vi "Test_LaunchHierarchy_StopRootModel_ConfirmOrderlyShutdown.vi"(8 "error in (no error)":errorcluster, 11 "TestCase in":refnum<class "TestLaunchAndShutdown.lvclass">) -> (0 "error out":errorcluster, 3 "TestCase out":refnum<class "TestLaunchAndShutdown.lvclass">)   [LabVIEW 2020, in "TestLaunchAndShutdown.lvclass"]
uses:
  TestLaunchAndShutdown.lvclass
  TestLaunchAndShutdown.lvclass/TestLaunchAndShutdown.ctl
  24bf8875-c008-4f22-9bfa-88e42476d167.vi
  Source/IModel/IModel/IModel.lvclass
  <vilib>/ActorFramework/Actor/Actor.lvclass
  Source/Mediator/Mediator/Mediator.lvclass
  <vilib>/ActorFramework/Stop Msg/Stop Msg.lvclass
  modules/composed-event-logger/Source/String Control Sink/String Control Sink.lvclass
  modules/composed-event-logger/Source/Composed Log/Types/Log Level.ctl
  modules/composed-event-logger/Source/Composed Log/Composed Log.lvlib
  modules/composed-event-logger/Source/String Formats/String Expression Format/String Expression Format.lvclass
  Doubles/RootModelNotifiesWhenStopped/RootModelNotifiesWhenStopped.lvclass
  C:/Git/mva-core/Source/RootModel/RootModel/RootModel.lvclass
  C:/Git/mva-core/Source/IModel/IModel/IModel.lvclass
  C:/Git/mva-core/Source/IObserver/IObserver/IObserver.lvclass
  C:/Program Files (x86)/National Instruments/LabVIEW 2020/vi.lib/ActorFramework/Actor/Actor.lvclass
  C:/Git/mva-core/Test/Doubles/RootModelNotifiesWhenStopped/RootModelNotifiesWhenStopped.lvclass
  9235eea7-0b3a-4059-b346-9cf3c4f5aec4.vi
  C:/Git/mva-core/modules/composed-event-logger/Source/IStringFormat/IStringFormat.lvclass
  C:/Git/mva-core/modules/composed-event-logger/Source/String Formats/String Expression Format/String Expression Format.lvclass
panel:
  in  "String":string
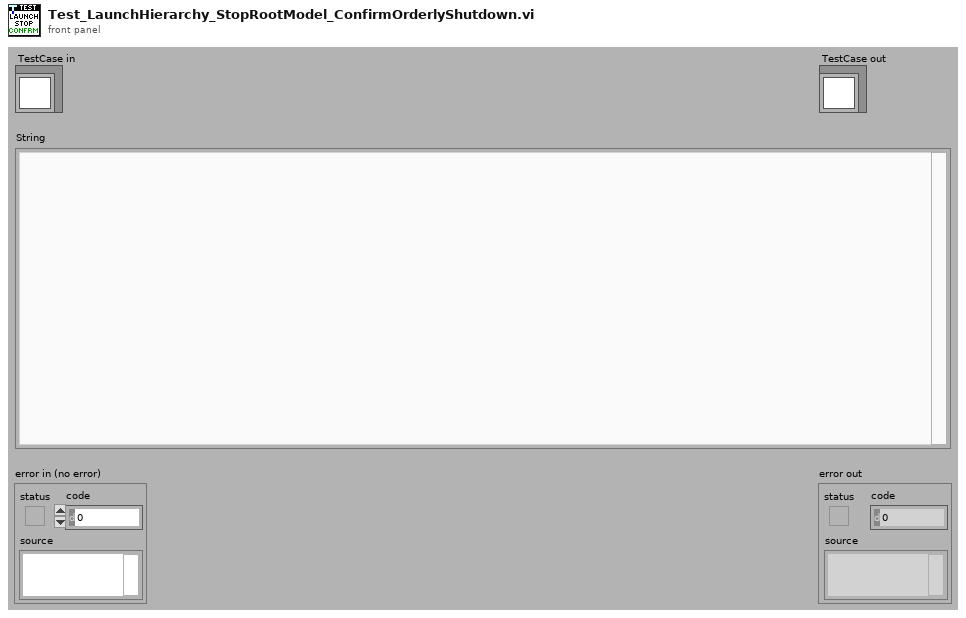
[diagram p1: front panel]
types:
  T1 = typedef "Composed Log.lvlib/Log Level.ctl" = enum16{"Debug", "Info", "Warning", "Error", "Critical"}
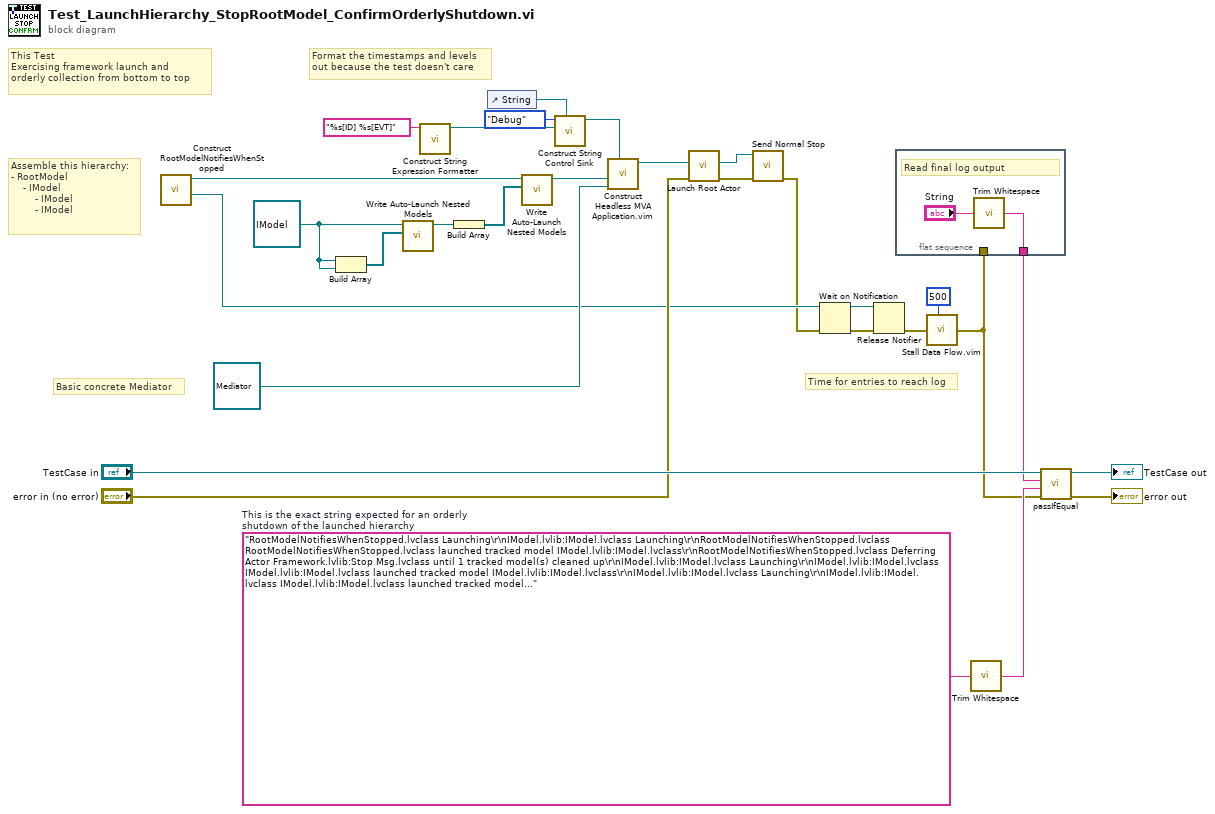
[diagram p0: block diagram]
diagram:
  w12 = "RootModelNotifiesWhenStopped.lvclass Launching\r\nIModel.lvlib:IModel.lvclass Launching\r\nRootModelNotifiesWhenStopped.lvclass RootModelNotifiesWhenStopped.lvclass launched tracked model IModel.lvlib:IModel.lvclass\r\nRootModelNotifiesWhenStopped.lvclass Deferring Actor Framework.lvlib:Stop Msg.lvclass until 1 tracked model(s) cleaned up\r\nIModel.lvlib:IModel.lvclass Launching\r\nIModel.lvlib:IModel.lvclass IModel.lvlib:IModel.lvclass launched tracked model IModel.lvlib:IModel.lvclass\r\nIModel.lvlib:IModel.lvclass Launching\r\nIModel.lvlib:IModel.lvclass IModel.lvlib:IModel.lvclass launched tracked model IModel.lvlib:IModel.lvclass\r\nIModel.lvlib:IModel.lvclass Deferring Actor Framework.lvlib:Stop Msg.lvclass until 2 tracked model(s) cleaned up\r\nIModel.lvlib:IModel.lvclass Stopped with 0 nested actors (final code: 0)\r\nIModel.lvlib:IModel.lvclass Stopped with 0 nested actors (final code: 0)\r\nIModel.lvlib:IModel.lvclass IModel.lvlib:IModel.lvclass collected IModel.lvlib:IModel.lvclass (final code: 0)\r\nIModel.lvlib:IModel.lvclass IModel.lvlib:IModel.lvclass collected IModel.lvlib:IModel.lvclass (final code: 0)\r\nIModel.lvlib:IModel.lvclass All tracked models stopped\r\nIModel.lvlib:IModel.lvclass Stopped with 0 nested actors (final code: 0)\r\nRootModelNotifiesWhenStopped.lvclass RootModelNotifiesWhenStopped.lvclass collected IModel.lvlib:IModel.lvclass (final code: 0)\r\nRootModelNotifiesWhenStopped.lvclass All tracked models stopped\r\nRootModelNotifiesWhenStopped.lvclass Stopped with 0 nested actors (final code: 0)"  # This is the exact string expected for an orderly shutdown of the launched hierarchy
  w19 = refnum<class "IModel.lvclass"> refnum ("IModel.lvlib:IModel.lvclass")
  # "This Test\nExercising framework launch and\norderly collection from bottom to top"
  # "Time for entries to reach log"
  # "Format the timestamps and levels\nout because the test doesn't care"
  # "Assemble this hierarchy:\n- RootModel\n    - IModel\n        - IModel\n        - IModel"
  # "Basic concrete Mediator"
  n1 = call "Construct RootModelNotifiesWhenStopped.vi"() -> ("Final Error Notifier"=w10:refnum<notifier>, "RootModelNotifiesWhenStopped out"=w11:refnum<class "RootModelNotifiesWhenStopped.lvclass">)  [unwired: 10 in]
  n2 = Build Array(w19, w19) -> (w20:refnum<class "IModel.lvclass">[])
  n3 = call "Write Auto-Launch Nested Models.vi"("Auto-Launch Nested Models"=w20, "IModel In"=w19) -> ("IModel Out"=w21:refnum<class "IModel.lvclass">)  [unwired: 9 in]
  n4 = call "Construct String Expression Formatter.vi"("Format Specifier"="%s[ID] %s[EVT]") -> ("String Expression Format out"=w14:refnum<class "String Expression Format.lvclass">)  [unwired: 9 in, 1 out]
  n5 = Build Array(w21) -> (w26:refnum<class "IModel.lvclass">[])
  n6 = control-ref of="String"() -> (w17:refnum<vi>)
  n7 = call "Write Auto-Launch Nested Models.vi"("Auto-Launch Nested Models"=w26, "IModel In"=w11) -> ("IModel Out"=w25:refnum<class "RootModelNotifiesWhenStopped.lvclass">)  [unwired: 9 in]
  n8 = call "Construct String Control Sink.vi"("Str Refnum"=w17, "LogFormat"=w14, "LogLevel"=Log_Level."Debug") -> ("String Control Sink out"=w18:refnum<class "String Control Sink.lvclass">)  [unwired: 8 in]
  n9 = call "Construct Headless MVA Application.vim"("Event Log Sink(s)"=w18, "Mediator Type"=refnum<class "Mediator.lvclass"> refnum ("Mediator.lvlib:Mediator.lvclass"), "RootModel in"=w25) -> ("RootModel out"=w24:refnum<class "RootModelNotifiesWhenStopped.lvclass">)  [unwired: 8 in]
  n10 = call <vilib>:"Launch Root Actor.vi"("error in (no error)"="error in (no error)", "Actor"=w24) -> ("error out"=w8:errorcluster, "Actor's Enqueuer"=w9:refnum<class "Message Enqueuer.lvclass">)  [unwired: 8 in]
  n11 = call <vilib>:"Send Normal Stop.vi"("error in (no error)"=w8, "Message Enqueuer"=w9) -> ("error out"=w5:errorcluster)  [unwired: 9 in]
  n12 = Wait on Notification(notifier=w10, error in (no error)=w5) -> (notifier out=w6:refnum<notifier>, error out=w7:errorcluster)  [unwired: 2 in, 2 out]
  n13 = Release Notifier(notifier=w6, error in (no error)=w7) -> (error out=w3:errorcluster)  [unwired: 1 in, 2 out]
  n14 = flat-sequence {
    tunnel: [w30] -> w16
    tunnel: w2 -> [_]
    frame #0 {
      # "Read final log output"
      n15 = call <vilib>:"Trim Whitespace.vi"("string"="String") -> ("trimmed string"=w30:string)  [unwired: 1 in]
    }
  }
  n16 = call "Stall Data Flow.vim"("value in"=w3, "milliseconds to wait"=u32 500) -> ("value out"=w2:errorcluster)  [unwired: 1 out]
  n17 = call <vilib>:"Trim Whitespace.vi"("string"=w12) -> ("trimmed string"=w4:string)  [unwired: 1 in]
  n18 = call-dynamic "passIfEqual.vi"("error in (no error)"=w2, "y"=w4, "x"=w16, "TestCase in"="TestCase in") -> ("error out"=→"error out":errorcluster, "TestCase out"=→"TestCase out":refnum<class "TestLaunchAndShutdown.lvclass">)  [unwired: 6 in]
